vi "华氏？ (2) Write.vi"(4 "error in (no error)":errorcluster, 5 "Value":bool, 6 "Container State":T2, 7 "Display State In":T1={"华氏?"=FALSE, "显示模式开关？"=TRUE}) -> (0 "error out":errorcluster, 3 "Display State Out":T1={"华氏?"=FALSE, "显示模式开关？"=TRUE})   [LabVIEW 2011, in "双模温度计2.xctl"]
uses:
  <vilib>/_xctls/Container State.ctl
  State.ctl
  <vilib>/_xctls/XControlSupport.lvlib
panel:
  # "Replace the Value Control below with a Control of desired type.\nDo not remove this Control or the others from the connector pane.\nDo not change the connector pane pattern.\nThe Value control should always be the third terminal from top on the input side in the connector pane."
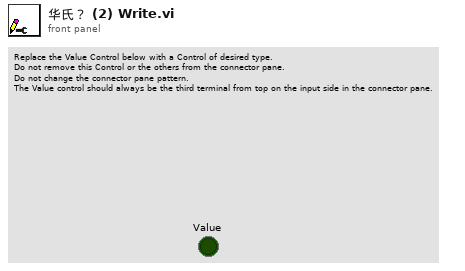
[diagram p1: front panel]
types:
  T1 = typedef "双模温度计2.xctl/State.ctl" = cluster{"华氏?":bool, "显示模式开关？":bool}
  T2 = typedef "XControlSupport.lvlib/Container State.ctl" = cluster{"Indicator?":bool, "Run Mode?":bool, " Refnum":refnum<vi>}
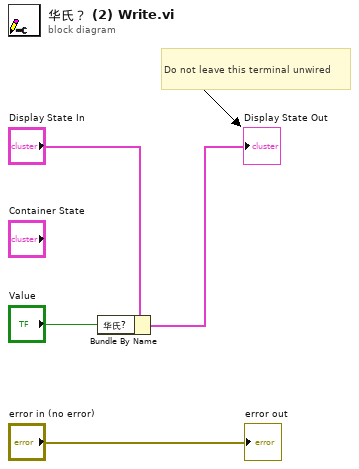
[diagram p0: block diagram]
diagram:
  # "Do not leave this terminal unwired"
  n1 = Bundle By Name(cluster="Display State In", "华氏?"="Value") -> (→"Display State Out":T1)
  "error out" <- "error in (no error)"
